vi "Get Data Path.vi"(8 "error in":errorcluster, 11 "File Observer in":refnum<class "File Observer.lvclass">) -> (0 "error out":errorcluster, 2 "path out":path, 3 "File Observer out":refnum<class "File Observer.lvclass">)   [LabVIEW 2015, in "File Observer.lvclass"]
doc: "This VI generates a data path to which files may be written. The default behavior is: \n\n1) Check to see if the top level data path (Top Data Path) exists; if it does not, then create it.\n2) Check to see if a folder to which we will write data in the Top Data Path exists; if it doesn't, create it. This folder is ultimately where the data files themselves will reside. The default behavior is to store data in folders based on the date, i.e. 'YYYYMMDD'.\n\nThis VI may be overridden to provide custom functionality for a particular application."
uses:
  File Observer.lvclass
  File Observer.lvclass/File Observer.ctl
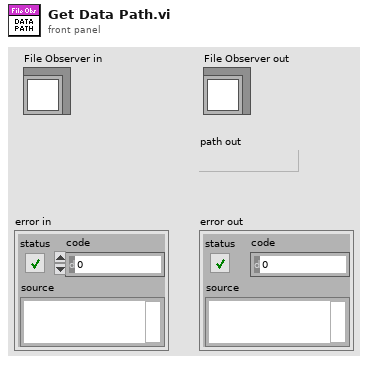
[diagram p1: front panel]
types:
  T1 = typedef "LVDateTimeRec.ctl" = cluster{"fractional second":dbl, "second":i32, "minute":i32, "hour":i32, "day of month":i32, "month":i32, "year":i32, "day of week":i32, "day of year":i32, "DST":i32}
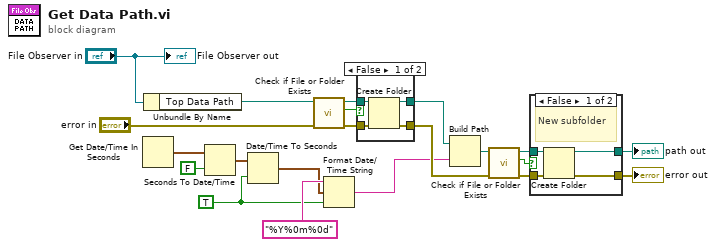
[diagram p0: block diagram]
diagram:
  w9 = TRUE ("is UTC (F)")
  n1 = Get Date/Time In Seconds() -> (seconds since 1Jan1904=w6:timestamp)
  n2 = Unbundle By Name("File Observer in") -> ("Top Data Path"=w1:path)
  n3 = Seconds To Date/Time(time stamp (now)=w6, to UTC (F)=FALSE) -> (date time rec=w8:T1)
  n4 = Date/Time To Seconds(1:w9, 2:w8) -> (0:w16:timestamp)
  n5 = call <vilib>:"Check if File or Folder Exists.vi"("error in (no error)"="error in", "path"=w1) -> ("error out"=w12:errorcluster, "file or folder exists?"=w20:bool, "dup path"=w11:path)  [unwired: 7 in]
  n6 = Format Date/Time String(time format string (%c)="%Y%0m%0d", seconds (now)=w16, UTC format=w9) -> (date/time string=w10:string)
  n7 = case shown="False" w20 {
    tunnel: w11 -> [w25 w27]
    tunnel: w12 -> [w24 w26]
    tunnel: [w23 w27] -> w13
    tunnel: [w22 w26] -> w14
    frame False {
      n8 = Create Folder(path (use dialog)=w25, error in=w24) -> (created path=w23:path, error out=w22:errorcluster)  [unwired: 1 in, 1 out]
    }
    frame True {
    }
  }
  n9 = Build Path(base path=w13, name or relative path=w10) -> (appended path=w5:path)
  n10 = call <vilib>:"Check if File or Folder Exists.vi"("error in (no error)"=w14, "path"=w5) -> ("error out"=w2:errorcluster, "file or folder exists?"=w4:bool, "dup path"=w3:path)  [unwired: 7 in]
  n11 = case "No directory with current date?\nMake one" shown="False" w4 {
    tunnel: w3 -> [w30 w33]
    tunnel: [w31 w33] -> w18
    tunnel: w2 -> [w29 w32]
    tunnel: [w28 w32] -> w19
    frame False {
      # "New subfolder"
      n12 = Create Folder(path (use dialog)=w30, error in=w29) -> (created path=w31:path, error out=w28:errorcluster)  [unwired: 1 in, 1 out]
    }
    frame True {
      # "Use current sub folder"
    }
  }
  "error out" <- w19
  "path out" <- w18
  "File Observer out" <- "File Observer in"
